vi "Select HDF5 Dialog (Object Only).vi"(0 "HDF5 File Ref":T2, 2 "Item Filters":T4 {"Object Types (any)" items=["H5G_UNKNOWN"=-1, "H5G_GROUP"=0, "H5G_DATASET"=1, "H5G_TYPE"=2, "H5G_LINK"=3, "H5G_UDLINK"=4]}, 7 "Initial Object Path":string, 9 "File Path Visible":bool, 11 "error in":errorcluster, 12 "Object Operation Mode":T1=enum."open or create", 13 "Window":T6={"Behavior"=enum."Modal", "Position"={"Left"=0, "Top"=0, "Right"=600, "Bottom"=400}, "Center"=TRUE, "Title"="Select an HDF5 Object"}) -> (4 "HDF5 File Ref out":T2, 8 "Object Path out":string, 10 "OK?":bool, 14 "Object operation out":T7(ring), 15 "error out":errorcluster)   [LabVIEW 2017]
doc: "Displays a dialog prompting the user to select a dataset, datatype,\n or group from an HDF5 file."
uses:
  <vilib>/Utility/miscctls.llb/LVRectTypeDef.ctl
  <vilib>/UPVI/lvhdf5/group.llb/H5G_obj_t.ctl
  <vilib>/UPVI/lvhdf5/library.llb/HDF5 Ref.ctl
  <vilib>/UPVI/lvhdf5/dataset.llb/LVH5D Operation.ctl
  <vilib>/UPVI/lvhdf5/file.llb/LVH5F Operation.ctl
panel:
  # "LVHDF5 Toolkit\nCopyright (c) 2005-2013 by Jason D. Sommerville\nCopyright (c) 2014 by UPVI, LLC.\n\nThis use and distribution of this file is governed by the terms found in \nLICENSE.txt distributed with this toolkit and installed at\n <user.lib>\\_lvhdf5\\LICENSE.txt"
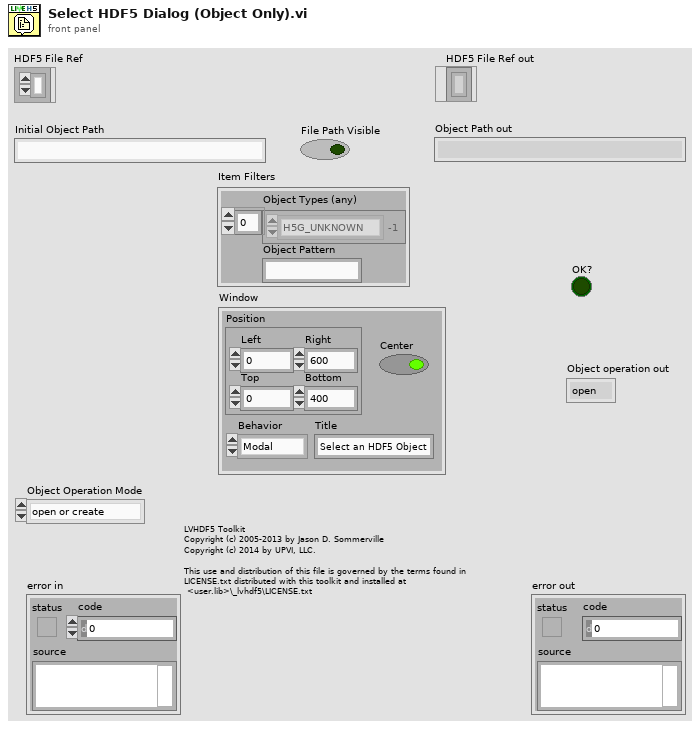
[diagram p1: front panel]
types:
  T1 = typedef "LVH5D Operation.ctl" = enum16{"open", "replace", "create", "open or create", "create or replace", "create or replace with confirmation"}
  T2 = typedef "HDF5 Ref.ctl" = refnum<k1>
  T3 = typedef "H5G_obj_t.ctl" = i32
  T4 = cluster{"Object Types (any)":T3[], "Object Pattern":string}
  T5 = typedef "LVRectTypeDef.ctl" = cluster{"Left":i16, "Top":i16, "Right":i16, "Bottom":i16}
  T6 = cluster{"Behavior":enum32{"Invalid", "Default", "Floating", "Floating/Auto-Hide", "Modal"}, "Position":T5, "Center":bool, "Title":string}
  T7 = enum16{"open", "replace", "create", "open or create", "replace or create", "replace or create with confirmation"}
  T8 = typedef "LVH5F Operation.ctl" = enum16{"open", "open or create", "create or replace", "create or replace (with confirmation)", "create", "open (read only)"}
  T9 = cluster{"File Mode--ignored":T8, "Object Operation Mode":T1}
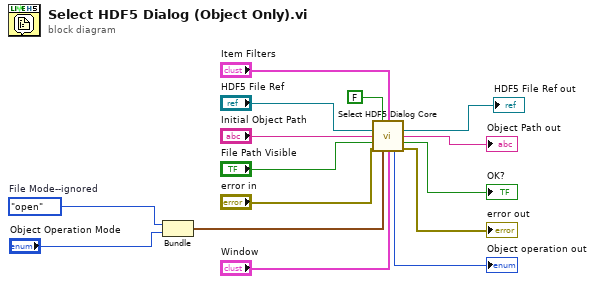
[diagram p0: block diagram]
diagram:
  w3 = LVH5F_Operation."open"  # File Mode--ignored
  n1 = Bundle("File Mode--ignored"=w3, "Object Operation Mode"="Object Operation Mode") -> (w1:T9)  [unwired: 1 in]
  n2 = call <vilib>:"Select HDF5 Dialog Core.vi"("Close HDF5 File?"=FALSE, "Item Filters"="Item Filters", "HDF5 File Ref"="HDF5 File Ref", "Initial Object Path"="Initial Object Path", "Path visible"="File Path Visible", "error in"="error in", "Operation Modes"=w1, "Window"="Window") -> ("HDF5 File Ref out"=→"HDF5 File Ref out":T2, "Object Path out"=→"Object Path out":string, "OK?"=→"OK?":bool, "Object operation out"=→"Object operation out":T7, "error out"=→"error out":errorcluster)  [unwired: 2 in, 1 out]
